vi "Fly.vi"(8 "error in (no error)":errorcluster, 11 "MallardDuck in":refnum<class "MallardDuck.lvclass">) -> (0 "error out":errorcluster, 2 "Fly":string, 3 "MallardDuck out":refnum<class "MallardDuck.lvclass">)   [LabVIEW 2013, in "MallardDuck.lvclass"]
uses:
  MallardDuck.lvclass
  Duck.lvclass/Duck.lvclass
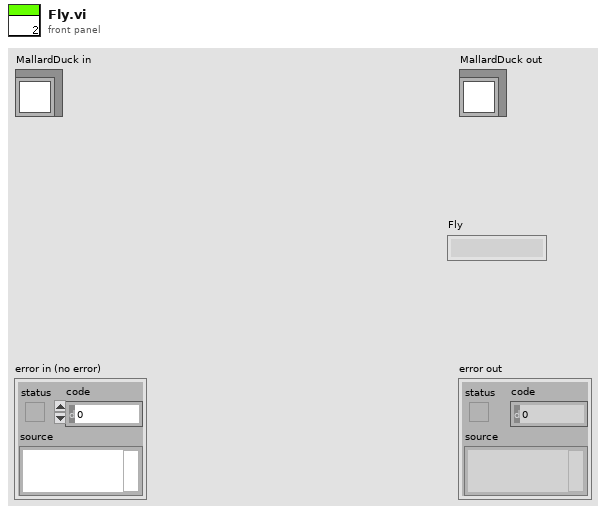
[diagram p1: front panel]
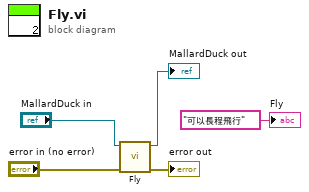
[diagram p0: block diagram]
diagram:
  n1 = call-parent "Fly.vi"("error in (no error)"="error in (no error)", "Duck in"="MallardDuck in") -> ("error out"=→"error out":errorcluster, "Duck out"=→"MallardDuck out":refnum<class "MallardDuck.lvclass">)  [unwired: 7 in, 1 out]
  "Fly" <- "可以長程飛行" ("Fly")
